vi "test Float Data Integrity.vi"(8 "error in (no error)":errorcluster, 11 "TestCase in":refnum<class "TestCase.lvclass">) -> (0 "error out":errorcluster, 3 "TestCase out":refnum<class "TestCase.lvclass">)   [LabVIEW 2017, in "Pointer Tests.lvlib" / "Data Manipulation Tests.lvclass"]
uses:
  Data Manipulation Tests.lvclass
  <vilib>/addons/_JKI Toolkits/VI Tester/TestCase.llb/TestCase.lvclass
  Source/Classes/Pointer/Public/New/New (4B).vi
  Source/Classes/Pointer/Public/Write/Write (1D SGL).vi
  Source/Classes/Pointer/Public/New/New (8B).vi
  Source/Classes/Pointer/Public/Write/Write (1D DBL).vi
  Source/Classes/Pointer/Public/Write/Write (0D SGL).vi
  Source/Classes/Pointer/Public/Write/Write (0D DBL).vi
  Source/Classes/Pointer/Pointer.lvclass
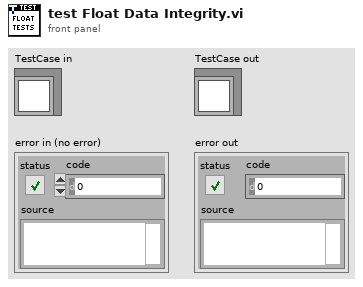
[diagram p1: front panel]
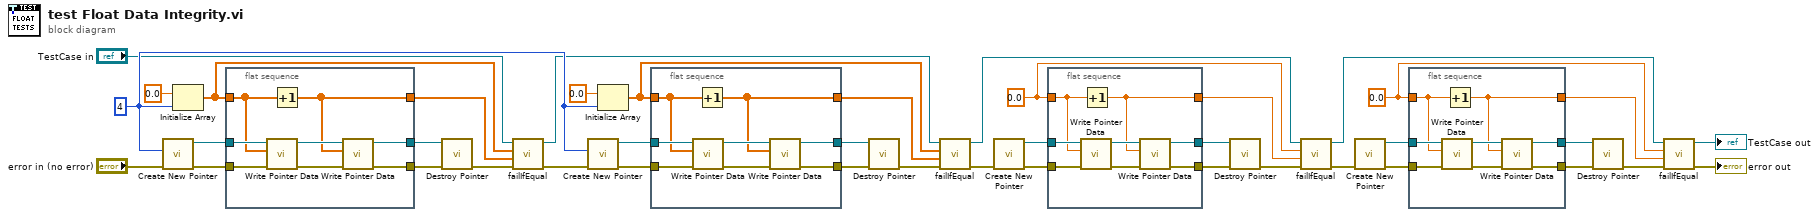
[diagram p0: block diagram]
diagram:
  w35 = u64 4 ("count (1)")
  w14 = 0.0 ("value")
  w3 = sgl 0.0 ("value")
  n1 = call-poly "Create New Pointer.vi"("error in (no error)"="error in (no error)", "count (1)"=w35) -> ("error out"=w29:errorcluster, "Pointer"=w26:refnum<class "Pointer.lvclass">)  [unwired: 8 in]
  n2 = Initialize Array(sgl 0.0 ("element"), w35) -> (w32:sgl[])
  n3 = flat-sequence {
    tunnel: w26 -> [w49]
    tunnel: [w47] -> w27
    tunnel: [w46] -> w28
    tunnel: w29 -> [w44]
    tunnel: w32 -> [w43]
    tunnel: [w42] -> w31
    frame #0 {
      n4 = call-poly "Write Pointer Data.vi"("error in (no error)"=w44, "buffer in"=w43, "Pointer in"=w49) -> ("error out"=w45:errorcluster, "Pointer out"=w48:refnum<class "Pointer.lvclass">)  [unwired: 5 in, 2 out]
      n5 = Increment(x=w43) -> (x+1=w42:sgl[])
      n6 = call-poly "Write Pointer Data.vi"("error in (no error)"=w45, "buffer in"=w42, "Pointer in"=w48) -> ("error out"=w46:errorcluster, "Pointer out"=w47:refnum<class "Pointer.lvclass">)  [unwired: 5 in, 2 out]
    }
  }
  n7 = call "Destroy Pointer.vi"("error in (no error)"=w28, "Pointer in"=w27) -> ("error out"=w30:errorcluster)  [unwired: 8 in, 1 out]
  n8 = call-dynamic "failIfEqual.vi"("error in (no error)"=w30, "y"=w31, "x"=w32, "TestCase in"="TestCase in") -> ("error out"=w18:errorcluster, "TestCase out"=w19:refnum<class "TestCase.lvclass">)  [unwired: 6 in]
  n9 = call-poly "Create New Pointer.vi"("error in (no error)"=w18, "count (1)"=w35) -> ("error out"=w22:errorcluster, "Pointer"=w25:refnum<class "Pointer.lvclass">)  [unwired: 8 in]
  n10 = Initialize Array(0.0 ("value"), w35) -> (w36:dbl[])
  n11 = flat-sequence {
    tunnel: w25 -> [w57]
    tunnel: [w55] -> w24
    tunnel: [w54] -> w23
    tunnel: w22 -> [w52]
    tunnel: w36 -> [w51]
    tunnel: [w50] -> w20
    frame #0 {
      n12 = call-poly "Write Pointer Data.vi"("error in (no error)"=w52, "buffer in"=w51, "Pointer in"=w57) -> ("error out"=w53:errorcluster, "Pointer out"=w56:refnum<class "Pointer.lvclass">)  [unwired: 5 in, 2 out]
      n13 = Increment(x=w51) -> (x+1=w50:dbl[])
      n14 = call-poly "Write Pointer Data.vi"("error in (no error)"=w53, "buffer in"=w50, "Pointer in"=w56) -> ("error out"=w54:errorcluster, "Pointer out"=w55:refnum<class "Pointer.lvclass">)  [unwired: 5 in, 2 out]
    }
  }
  n15 = call "Destroy Pointer.vi"("error in (no error)"=w23, "Pointer in"=w24) -> ("error out"=w21:errorcluster)  [unwired: 8 in, 1 out]
  n16 = call-dynamic "failIfEqual.vi"("error in (no error)"=w21, "y"=w20, "x"=w36, "TestCase in"=w19) -> ("error out"=w38:errorcluster, "TestCase out"=w41:refnum<class "TestCase.lvclass">)  [unwired: 6 in]
  n17 = call-poly "Create New Pointer.vi"("error in (no error)"=w38) -> ("error out"=w5:errorcluster, "Pointer"=w8:refnum<class "Pointer.lvclass">)  [unwired: 9 in]
  n18 = flat-sequence {
    tunnel: w8 -> [w65]
    tunnel: [w63] -> w7
    tunnel: [w62] -> w6
    tunnel: w5 -> [w60]
    tunnel: w3 -> [w59]
    tunnel: [w58] -> w2
    frame #0 {
      n19 = call-poly "Write Pointer Data.vi"("error in (no error)"=w60, "value"=w59, "Pointer in"=w65) -> ("error out"=w61:errorcluster, "Pointer out"=w64:refnum<class "Pointer.lvclass">)  [unwired: 5 in, 2 out]
      n20 = Increment(x=w59) -> (x+1=w58:sgl)
      n21 = call-poly "Write Pointer Data.vi"("error in (no error)"=w61, "value"=w58, "Pointer in"=w64) -> ("error out"=w62:errorcluster, "Pointer out"=w63:refnum<class "Pointer.lvclass">)  [unwired: 5 in, 2 out]
    }
  }
  n22 = call "Destroy Pointer.vi"("error in (no error)"=w6, "Pointer in"=w7) -> ("error out"=w4:errorcluster)  [unwired: 8 in, 1 out]
  n23 = call-dynamic "failIfEqual.vi"("error in (no error)"=w4, "y"=w2, "x"=w3, "TestCase in"=w41) -> ("error out"=w17:errorcluster, "TestCase out"=w16:refnum<class "TestCase.lvclass">)  [unwired: 6 in]
  n24 = call-poly "Create New Pointer.vi"("error in (no error)"=w17) -> ("error out"=w12:errorcluster, "Pointer"=w9:refnum<class "Pointer.lvclass">)  [unwired: 9 in]
  n25 = flat-sequence {
    tunnel: w9 -> [w73]
    tunnel: [w71] -> w10
    tunnel: [w70] -> w11
    tunnel: w12 -> [w68]
    tunnel: w14 -> [w67]
    tunnel: [w66] -> w15
    frame #0 {
      n26 = call-poly "Write Pointer Data.vi"("error in (no error)"=w68, "value"=w67, "Pointer in"=w73) -> ("error out"=w69:errorcluster, "Pointer out"=w72:refnum<class "Pointer.lvclass">)  [unwired: 5 in, 2 out]
      n27 = Increment(x=w67) -> (x+1=w66:dbl)
      n28 = call-poly "Write Pointer Data.vi"("error in (no error)"=w69, "value"=w66, "Pointer in"=w72) -> ("error out"=w70:errorcluster, "Pointer out"=w71:refnum<class "Pointer.lvclass">)  [unwired: 5 in, 2 out]
    }
  }
  n29 = call "Destroy Pointer.vi"("error in (no error)"=w11, "Pointer in"=w10) -> ("error out"=w13:errorcluster)  [unwired: 8 in, 1 out]
  n30 = call-dynamic "failIfEqual.vi"("error in (no error)"=w13, "y"=w15, "x"=w14, "TestCase in"=w16) -> ("error out"=→"error out":errorcluster, "TestCase out"=→"TestCase out":refnum<class "TestCase.lvclass">)  [unwired: 6 in]
